vi "StandaloneManualValveControl.vi"() -> ()   [LabVIEW 2018]
uses:
  <vilib>/MakerHub/LINX/Public/Peripherals/Digital/Digital Write N Chans.vi
  <vilib>/MakerHub/LINX/Private/Local IO/LinxDigitalWrite.vi
  <vilib>/MakerHub/LINX/Public/Utilities/Check Channel.vi
  <vilib>/MakerHub/LINX/Public/Utilities/Open Serial.vi
  <vilib>/MakerHub/LINX/Private/Utilties/Generate Error.vi
  <vilib>/MakerHub/LINX/LMH-LINX.lvlib
panel:
  out "Error Out":errorcluster
  out "Device Name":string
  in  "error in (no error)":errorcluster
  in  "VISA resource name":refnum<visa-resource-name>
  in  "Manually controlled Valves":u8[](array[numeric])
  out "Open?":bool
  in  "Manual Open":bool
  in  "stop":bool
  # "ALWAYS TERMINATE THE\nPROGRAM WITH THIS STOP BUTTON!"
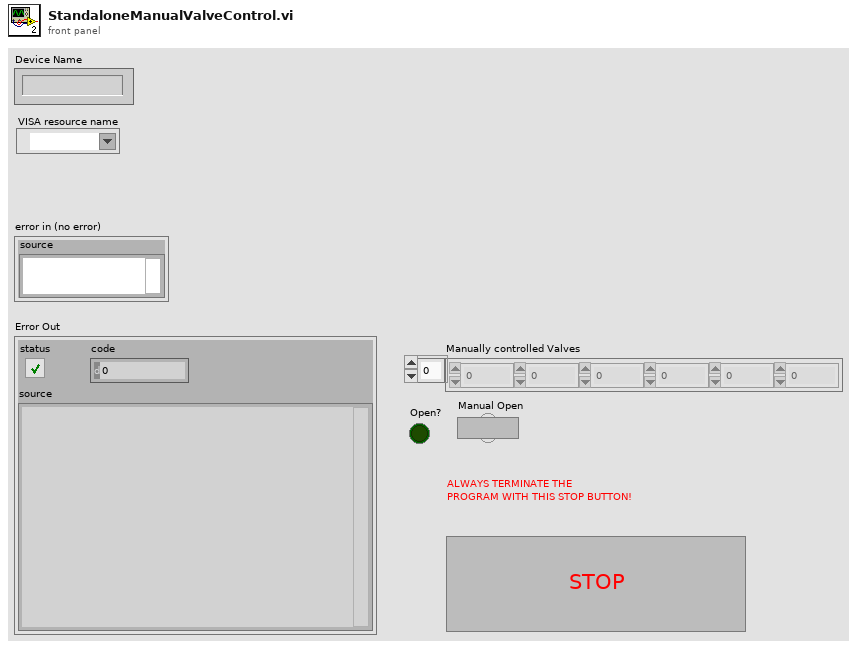
[diagram p1: front panel]
types:
  T1 = typedef "LMH-LINX.lvlib/LINX Ref.ctl" = cluster{"IO":T2, "Interface":T3, "LINX Device Config":T4}
  T2 = typedef "LMH-LINX.lvlib/Platform.ctl" = enum16{"Remote", "Local"}
  T3 = typedef "LMH-LINX.lvlib/Interface.ctl" = enum16{"Serial", "TCP"}
  T4 = typedef "LMH-LINX.lvlib/Device.lvlib/LINX Device Config.ctl" = cluster{"Interface":T3, "COM Port":refnum<visa-resource-name>, "TCP Configuration":T5, "Device Family":u8, "Device ID":u8, "Device Name":string, "TCP Ref":refnum<k5>, "Channels":T6}
  T5 = typedef "LMH-LINX.lvlib/Device.lvlib/TCP Config.ctl" = cluster{"IP Address":string, "Port":u16}
  T6 = typedef "LMH-LINX.lvlib/Channels.ctl" = cluster{"DI":u8[], "DO":u8[], "AI":u8[], "AO":u8[], "PWM":u8[], "QE":u8[], "UART":u8[], "I2C 2":u8[], "SPI":u8[], "CAN":u8[], "Servo":u8[], "AI Ref (V)":dbl, "AI Resolution (Bits)":u8, "AO Ref (V)":dbl, "AO Resolution (Bits)":u8}
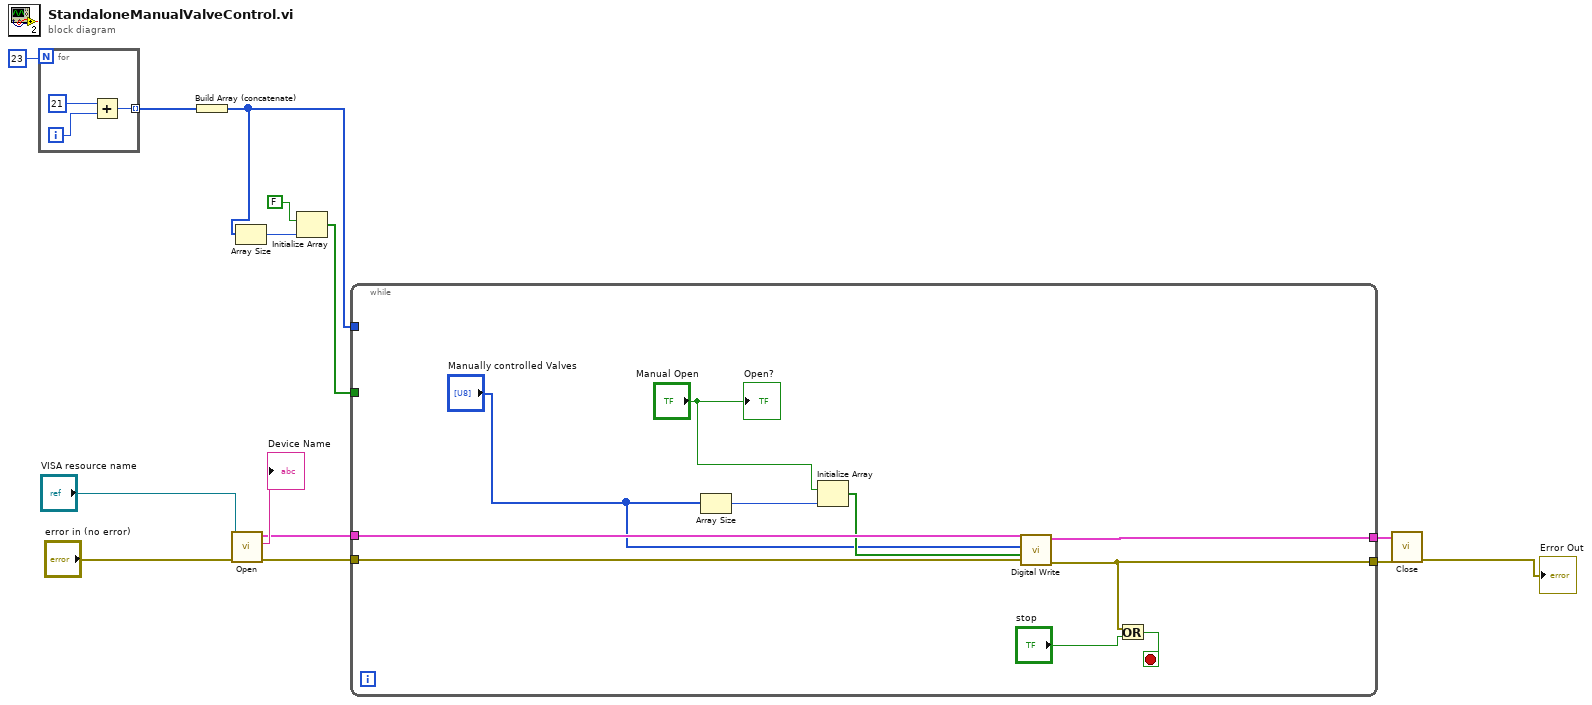
[diagram p0: block diagram]
diagram:
  n1 = for {
    N: 23 -> [_]
    tunnel: [w15] -> w5 mode=indexing
    i -> [w17]
    n2 = Add(x=21, y=w17) -> (x+y=w15:i32)
  }
  n3 = Build Array (concatenate)(w5) -> (w4:i32[])
  n4 = call-poly <vilib>:"Open.vi"("Error In"="error in (no error)", "Serial Port"="VISA resource name") -> ("Error Out"=w7:errorcluster, "Device Name"=→"Device Name":string, "LINX Resource"=w8:T1)  [unwired: 7 in]
  n5 = Array Size(array=w4) -> (size(s)=w3:i32)
  n6 = Initialize Array(FALSE, w3) -> (w1:bool[])
  n7 = while {
    tunnel: w8 -> [w27]
    tunnel: [w26] -> w10
    tunnel: w7 -> [w25]
    tunnel: [w22] -> w9
    tunnel: w4 -> [_]
    tunnel: w1 -> [_]
    stop <- w23 stop-if-true
    n8 = Array Size(array="Manually controlled Valves") -> (size(s)=w21:i32)
    n9 = Initialize Array("Manual Open", w21) -> (w20:bool[])
    n10 = call-poly <vilib>:"Digital Write.vi"("Error In"=w25, "Values"=w20, "DO Channels"="Manually controlled Valves", "LINX Resource"=w27) -> ("Error Out"=w22:errorcluster, "LINX Resource"=w26:T1)  [unwired: 6 in]
    n11 = Or(x=w22, y="stop") -> (x .or. y?=w23:bool)
    "Open?" <- "Manual Open"
  }
  n12 = call <vilib>:"Close.vi"("Error In"=w9, "LINX Resource"=w10) -> ("Error Out"=→"Error Out":errorcluster)  [unwired: 9 in]
